vi "Write Frame.vi"(8 "error in (no error)":errorcluster, 10 "ARGB Image in":T1, 11 "Writer (ARGB) in":refnum<class "Writer (ARGB).lvclass">) -> (0 "error out":errorcluster, 3 "Writer (ARGB)":refnum<class "Writer (ARGB).lvclass">)   [LabVIEW 2020, in "video_io.lvlib" / "Writer (ARGB).lvclass"]
uses:
  Writer (ARGB).lvclass
  image/ARGB Image.ctl
  Writer (ARGB).lvclass/Writer (ARGB).ctl
  0e3f49b0-4303-46d3-b8ab-944fedc4b55e.vi
  <vilib>/Utility/error.llb/Error Cluster From Error Code.vi
  image/image.lvlib
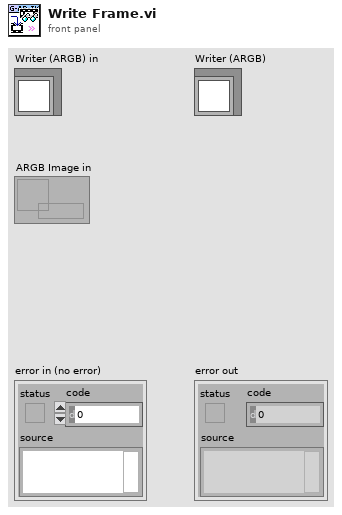
[diagram p1: front panel]
types:
  T1 = typedef "image.lvlib/ARGB Image.ctl" = refnum<data-value>
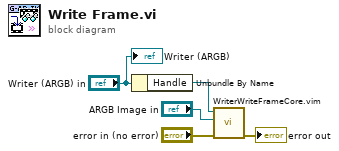
[diagram p0: block diagram]
diagram:
  n1 = Unbundle By Name("Writer (ARGB) in") -> ("Handle"=w4:refnum<data-value>)
  n2 = call "WriterWriteFrameCore.vim"("error in (no error)"="error in (no error)", "Greyscale Image"="ARGB Image in", "Handle"=w4) -> ("error out"=→"error out":errorcluster)  [unwired: 8 in]
  "Writer (ARGB)" <- "Writer (ARGB) in"
